vi "系统设置.vi"() -> ()   [LabVIEW 2016]
uses:
  <vilib>/Utility/miscctls.llb/LVPointTypeDef.ctl
  <vilib>/Utility/config.llb/Read Key (U32).vi
  <vilib>/Utility/config.llb/Write Key (I32).vi
  PLC/PLC.lvlib
  <vilib>/ptbypt/NI_PtbyPt.lvlib
  <vilib>/Utility/config.llb/NI_LVConfig.lvlib
panel:
  in  "采水模式":enum16{"使用采水泵", "不使用采水泵"}(ring)
  in  "运行模式":enum16{"维护模式", "常规模式", "应急模式", "质控模式"}(ring)
  in  "运行间隔":i16=4 min=1 max=24
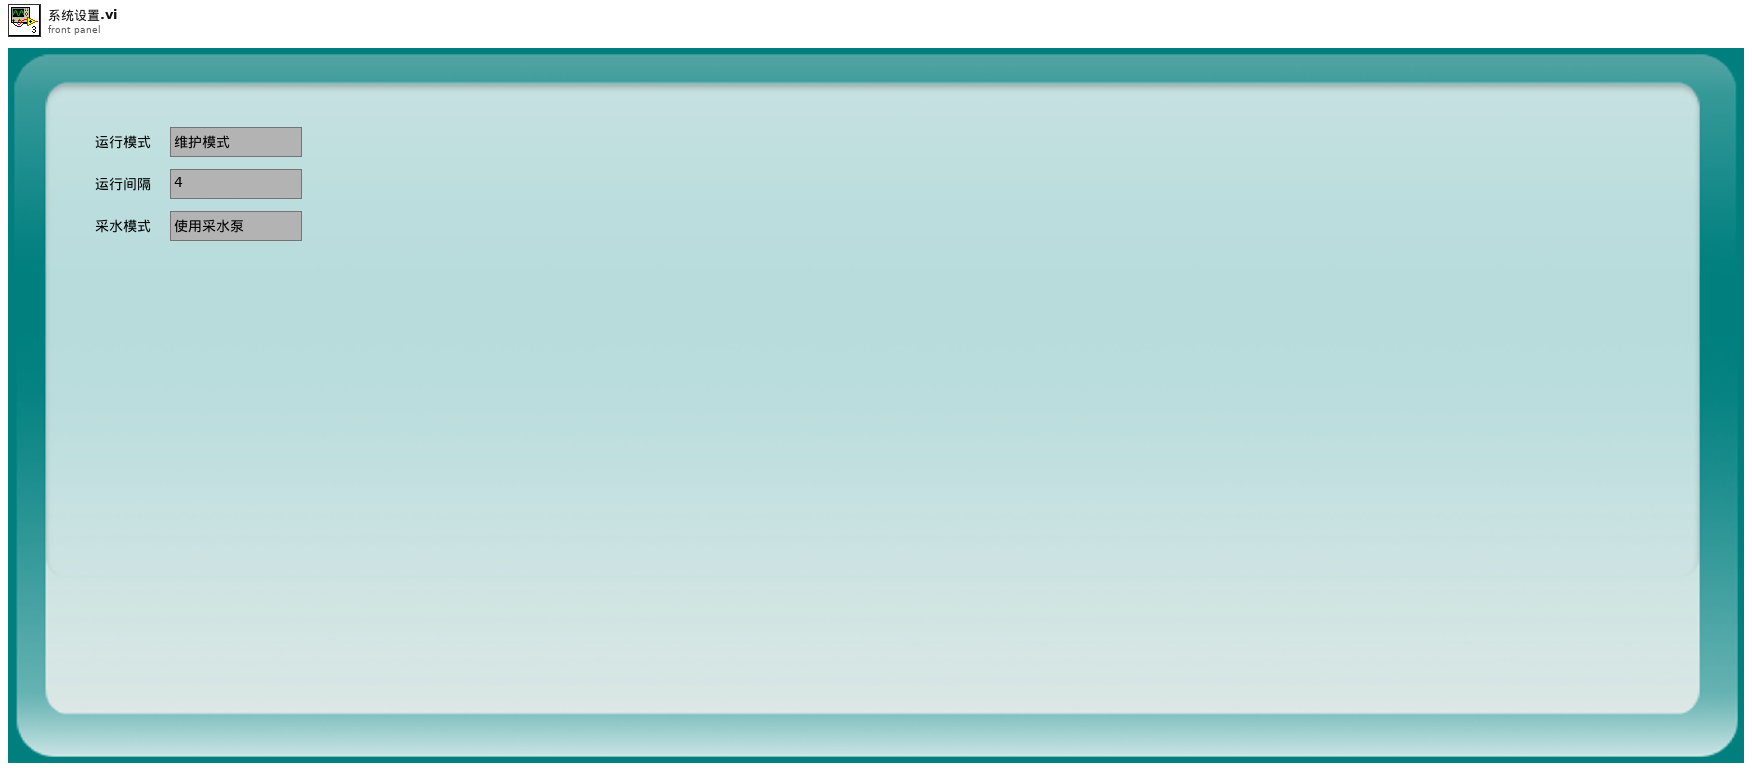
[diagram p1: front panel]
types:
  T1 = typedef "LVPointTypeDef.ctl" = cluster{"Horizontal":i16, "Vertical":i16}
  T2 = typedef "NI_LVConfig.lvlib/Config Data RefNum.ctl" = refnum<k1>
  T3 = cluster{"是否启用仪器":bool, "CODMn":cluster{"启动测量模式":cluster{"测量模式":enum16{"水样测量", "标样核查", "零点核查", "加标回收", "平行样", "校零", "校标"}}, "确定按钮":bool}, "采水模式":enum16{"使用采水泵", "不使用采水泵"}}
  T4 = enum16{"水样测量", "标样核查", "零点核查", "加标回收", "平行样", "校零", "校标"}
  T5 = typedef "LVDateTimeRec.ctl" = cluster{"秒数的小数部分":dbl, "秒":i32, "分":i32, "时":i32, "日":i32, "月":i32, "年":i32, "天数（周）":i32, "天数（年）":i32, "DST":i32}
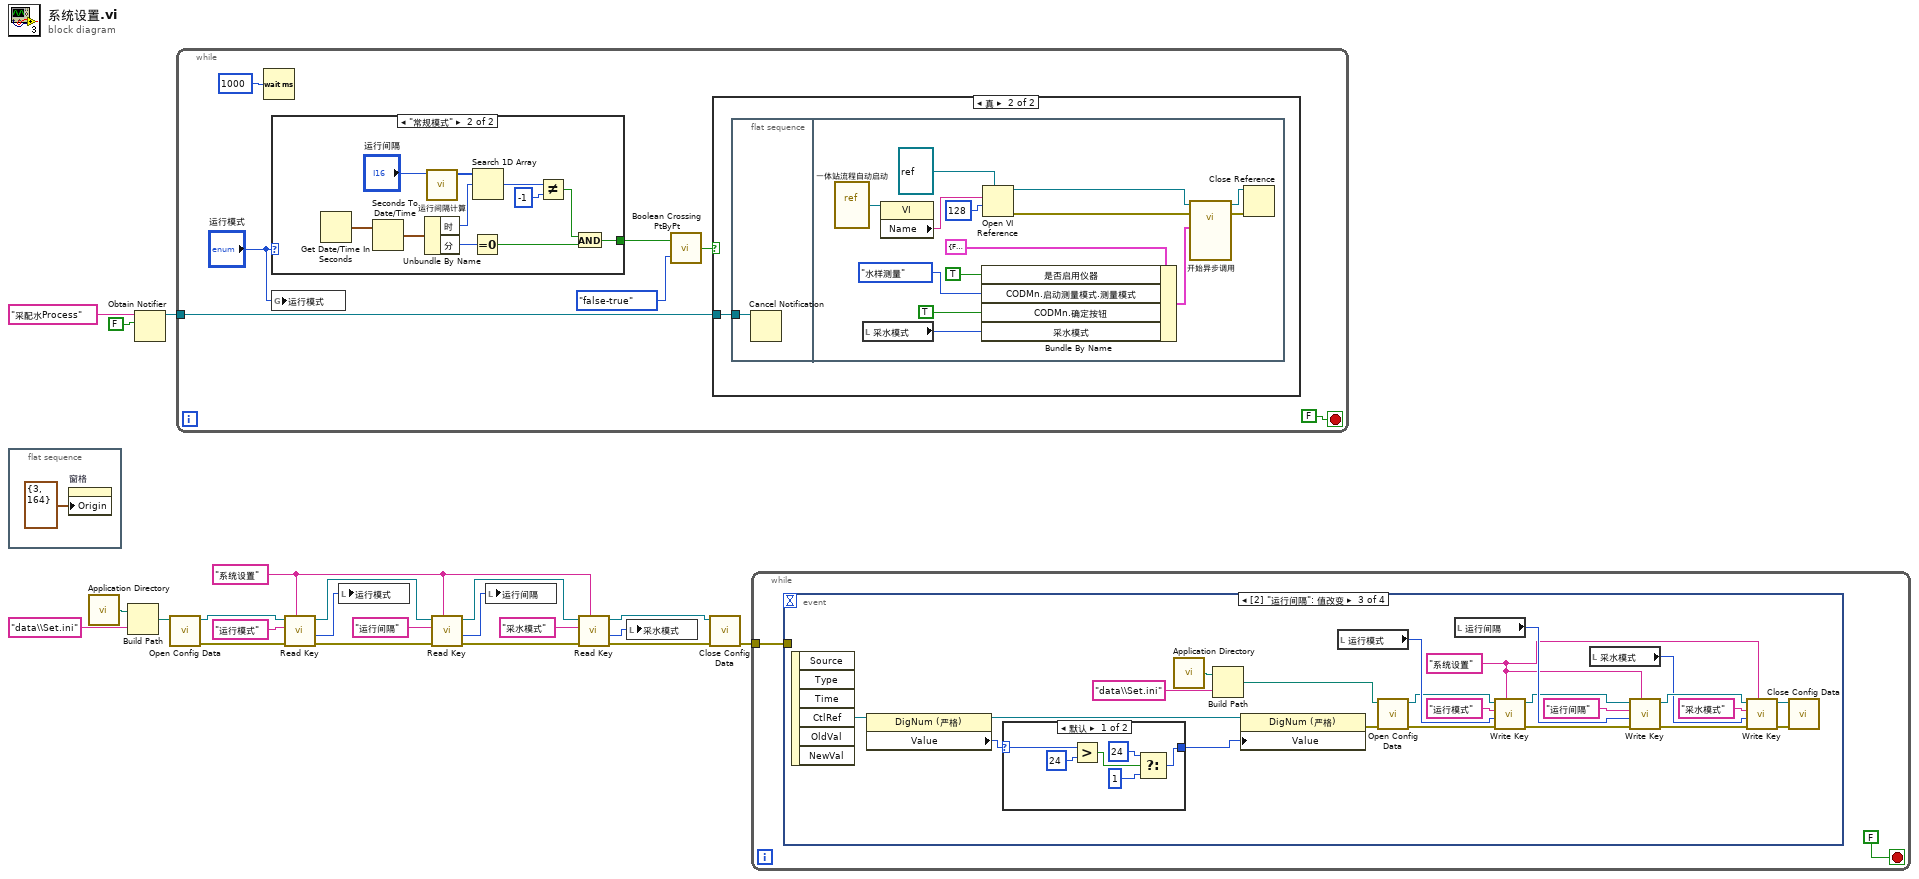
[diagram p0: block diagram]
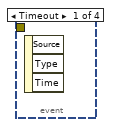
[diagram p4: hidden frame]
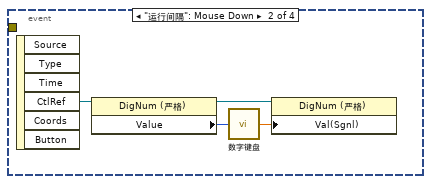
[diagram p5: hidden frame]
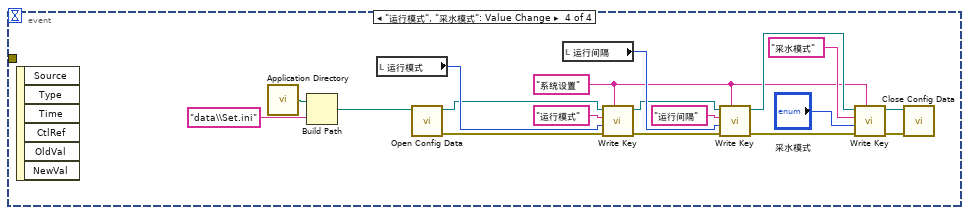
[diagram p7: hidden frame]
diagram:
  w3 = "系统设置" ("section")
  n1 = flat-sequence {
    frame #0 {
      n2 = property on="窗格" class="Pane"("Origin"=T1 {"Horizontal"=3, "Vertical"=164} ("原点")) -> ()  [unwired: 2 in, 2 out]
    }
  }
  n3 = call <vilib>:"Application Directory.vi"() -> ("Application Directory"=w17:path)
  n4 = Build Path(base path=w17, name or relative path="data\\Set.ini" ("名称或相对路径")) -> (appended path=w15:path)
  n5 = Obtain Notifier(name (unnamed)="采配水Process" ("名称（未命名）"), notification data type=FALSE) -> (notifier out=w20:refnum<notifier>)  [unwired: 2 in, 2 out]
  n6 = call <vilib>:"Open Config Data.vi"("configuration file path"=w15) -> ("error out"=w18:errorcluster, "refnum"=w19:T2)  [unwired: 8 in, 1 out]
  n7 = while {
    tunnel: w20 -> [w28]
    stop <- FALSE stop-if-true
    n8 = Wait (ms)(milliseconds to wait=u32 1000 ("等待时间（毫秒）")) -> ()  [unwired: 1 out]
    n9 = case shown="\"常规模式\"" "运行模式" {
      tunnel: [_ w47] -> w27
      frame "维护模式", Default {
      }
      frame "常规模式" {
        n10 = Get Date/Time In Seconds() -> (seconds since 1Jan1904=w56:timestamp)
        n11 = Seconds To Date/Time(time stamp (now)=w56) -> (date time rec=w55:T5)  [unwired: 1 in]
        n12 = Unbundle By Name(w55) -> ("时"=w52:i32, "分"=w54:i32)
        n13 = call "运行间隔计算.vi"("运行周期"="运行间隔") -> ("数组"=w53:i32[])  [unwired: 10 in]
        n14 = Equal To 0?(x=w54) -> (x = 0?=w48:bool)
        n15 = Search 1D Array(1D array=w53, element=w52) -> (index of element=w51:i32)  [unwired: 1 in]
        n16 = Not Equal?(x=w51, y=-1) -> (x != y?=w49:bool)
        n17 = And(x=w49, y=w48) -> (x .and. y?=w47:bool)
      }
    }
    n18 = global write "系统变量.vi" "运行模式"("运行模式") -> ()
    n19 = call <vilib>:"Boolean Crossing PtByPt.vi"("direction"=enum16{"either", "false-true", "true-false"}."false-true", "input"=w27) -> ("crossing"=w25:bool)  [unwired: 1 in]
    n20 = case shown="真" w25 {
      tunnel: w28 -> [_ w31]
      frame False {
      }
      frame True {
        n21 = flat-sequence {
          tunnel: w31 -> [w32]
          frame #0 {
            n22 = Cancel Notification(0:w32) -> ()  [unwired: 1 in, 3 out]
          }
          frame #1 {
            n23 = vi-ref "一体站流程自动启动.vi"() -> (w46:refnum<vi>)
            n24 = local read "采水模式"() -> (w34:enum16{"使用采水泵", "不使用采水泵"})
            n25 = property class="VI"(reference=w46) -> ("Name"=w45:string)  [unwired: 1 in, 2 out]
            n26 = Bundle By Name(cluster=T3 {"是否启用仪器"=FALSE, "CODMn"={"启动测量模式"={"测量模式"=enum."水样测量"}, "确定按钮"=FALSE}, "采水模式"=enum."使用采水泵"} ("参数"), "是否启用仪器"=TRUE, "CODMn.启动测量模式.测量模式"=T4."水样测量", "CODMn.确定按钮"=TRUE, "采水模式"=w34) -> (w33:T3)
            n27 = Open VI Reference(type specifier VI Refnum (for type only)=refnum<vi> refnum, vi path=w45, options=128 ("选项")) -> (vi reference=w43:refnum<vi>, error out=w40:errorcluster)  [unwired: 3 in]
            n28 = call-by-ref "开始异步调用"(reference=w43, error in=w40, "参数"=w33) -> (reference out=w41:refnum<vi>, error out=w39:errorcluster)  [unwired: 11 in]
            n29 = Close Reference(reference=w41, error in (no error)=w39) -> ()  [unwired: 1 out]
          }
        }
      }
    }
  }
  n30 = call-poly <vilib>:"Read Key.vi"("section"=w3, "error in (no error)"=w18, "key"="运行模式" ("section"), "refnum"=w19) -> ("error out"=w12:errorcluster, "value"=w14:u32, "refnum out"=w13:T2)  [unwired: 4 in, 1 out]
  n31 = local write "运行模式"(w14) -> ()
  n32 = call-poly <vilib>:"Read Key.vi"("section"=w3, "error in (no error)"=w12, "key"="运行间隔" ("section"), "refnum"=w13) -> ("error out"=w6:errorcluster, "value"=w9:u32, "refnum out"=w7:T2)  [unwired: 4 in, 1 out]
  n33 = local write "运行间隔"(w9) -> ()
  n34 = call-poly <vilib>:"Read Key.vi"("section"=w3, "error in (no error)"=w6, "key"="采水模式", "refnum"=w7) -> ("error out"=w4:errorcluster, "value"=w1:u32, "refnum out"=w5:T2)  [unwired: 4 in, 1 out]
  n35 = local write "采水模式"(w1) -> ()
  n36 = call <vilib>:"Close Config Data.vi"("error in (no error)"=w4, "refnum"=w5) -> ("error out"=w8:errorcluster)  [unwired: 8 in, 1 out]
  n37 = while {
    tunnel: w8 -> [w58]
    stop <- FALSE stop-if-true
    n38 = event shown="[2] \"运行间隔\": 值改变" {
      selector: _ -> [_ _ _ _]
      dyn-events: _ -> [_ _ _ _]
      timeout: _ -> [_ _ _ _]
      tunnel: w58 -> [_ _ _ _]
      event Timeout {
        n39 = event-data() -> ()  [unwired: 1 in, 3 out]
      }
      event "运行间隔": Mouse Down {
        n40 = event-data() -> ("CtlRef"=w60:refnum<vi>)  [unwired: 1 in, 5 out]
        n41 = property class="DigNum (严格)"(reference=w60) -> (reference out=w62:refnum<vi>, "Value"=w61:i16)  [unwired: 1 in, 1 out]
        n42 = call "数字键盘.vi"("OldNumber"=w61) -> ("NewNumber"=w63:sgl)
        n43 = property class="DigNum (严格)"(reference=w62, "Val(Sgnl)"=w63) -> ()  [unwired: 1 in, 2 out]
      }
      event "运行间隔": Value Change {
        w64 = "系统设置" ("section")
        n44 = event-data() -> ("CtlRef"=w86:refnum<vi>)  [unwired: 1 in, 5 out]
        n45 = property class="DigNum (严格)"(reference=w86) -> (reference out=w84:refnum<vi>, "Value"=w85:i16)  [unwired: 1 in, 1 out]
        n46 = case shown="默认" w85 {
          selector: w85 -> [w89 w93]
          tunnel: [w88 w93] -> w83
          frame Default {
            n47 = Greater?(x=w89, y=i16 24) -> (0:w91:bool)
            n48 = Select(t=i16 24 ("y"), s=w91, f=i16 1) -> (s? t:f=w88:i16)
          }
          frame 1..24 {
          }
        }
        n49 = call <vilib>:"Application Directory.vi"() -> ("Application Directory"=w78:path)
        n50 = Build Path(base path=w78, name or relative path="data\\Set.ini" ("名称或相对路径")) -> (appended path=w76:path)
        n51 = property class="DigNum (严格)"(reference=w84, "Value"=w83) -> (error out=w71:errorcluster)  [unwired: 1 in, 1 out]
        n52 = local read "运行模式"() -> (w81:enum16{"维护模式", "常规模式", "应急模式", "质控模式"})
        n53 = call <vilib>:"Open Config Data.vi"("error in (no error)"=w71, "configuration file path"=w76) -> ("error out"=w79:errorcluster, "refnum"=w80:T2)  [unwired: 7 in, 1 out]
        n54 = local read "运行间隔"() -> (w82:i16)
        n55 = call-poly <vilib>:"Write Key.vi"("section"=w64, "error in (no error)"=w79, "value"=w81, "key"="运行模式" ("section"), "refnum"=w80) -> ("error out"=w74:errorcluster, "refnum out"=w75:T2)  [unwired: 4 in, 1 out]
        n56 = local read "采水模式"() -> (w65:enum16{"使用采水泵", "不使用采水泵"})
        n57 = call-poly <vilib>:"Write Key.vi"("section"=w64, "error in (no error)"=w74, "value"=w82, "key"="运行间隔" ("section"), "refnum"=w75) -> ("error out"=w67:errorcluster, "refnum out"=w69:T2)  [unwired: 4 in, 1 out]
        n58 = call-poly <vilib>:"Write Key.vi"("section"=w64, "error in (no error)"=w67, "value"=w65, "key"="采水模式", "refnum"=w69) -> ("error out"=w66:errorcluster, "refnum out"=w68:T2)  [unwired: 4 in, 1 out]
        n59 = call <vilib>:"Close Config Data.vi"("error in (no error)"=w66, "refnum"=w68) -> ()  [unwired: 8 in, 2 out]
      }
      event "运行模式", "采水模式": Value Change {
        w94 = "系统设置" ("section")
        n60 = event-data() -> ()  [unwired: 1 in, 6 out]
        n61 = call <vilib>:"Application Directory.vi"() -> ("Application Directory"=w107:path)
        n62 = Build Path(base path=w107, name or relative path="data\\Set.ini" ("名称或相对路径")) -> (appended path=w105:path)
        n63 = local read "运行模式"() -> (w110:enum16{"维护模式", "常规模式", "应急模式", "质控模式"})
        n64 = call <vilib>:"Open Config Data.vi"("configuration file path"=w105) -> ("error out"=w108:errorcluster, "refnum"=w109:T2)  [unwired: 8 in, 1 out]
        n65 = local read "运行间隔"() -> (w111:i16)
        n66 = call-poly <vilib>:"Write Key.vi"("section"=w94, "error in (no error)"=w108, "value"=w110, "key"="运行模式" ("section"), "refnum"=w109) -> ("error out"=w103:errorcluster, "refnum out"=w104:T2)  [unwired: 4 in, 1 out]
        n67 = call-poly <vilib>:"Write Key.vi"("section"=w94, "error in (no error)"=w103, "value"=w111, "key"="运行间隔" ("section"), "refnum"=w104) -> ("error out"=w96:errorcluster, "refnum out"=w98:T2)  [unwired: 4 in, 1 out]
        n68 = call-poly <vilib>:"Write Key.vi"("section"=w94, "error in (no error)"=w96, "value"="采水模式", "key"="采水模式", "refnum"=w98) -> ("error out"=w95:errorcluster, "refnum out"=w97:T2)  [unwired: 4 in, 1 out]
        n69 = call <vilib>:"Close Config Data.vi"("error in (no error)"=w95, "refnum"=w97) -> ()  [unwired: 8 in, 2 out]
      }
    }
  }
